vi "Write Configuration File.vi"(8 "error in (no error)":errorcluster, 11 "Example Instrument in":refnum<class "Instrument.LN2.lvclass">) -> (0 "error out":errorcluster, 3 "Example Instrument out":refnum<class "Instrument.LN2.lvclass">)   [LabVIEW 2019, in "Instrument.LN2.lvclass"]
uses:
  Instrument.LN2.lvclass
  <userlib>/LevyLab/Instrument Framework/Instrument Types/VSource/Instrument.VSource.lvclass
  <userlib>/LevyLab/Instrument Framework/SMOs/Configuration/Configuration.lvclass
  <userlib>/LevyLab/Instrument Framework/SMOs/Instrument/Instrument.lvclass
  C:/Program Files (x86)/National Instruments/LabVIEW 2019/user.lib/LevyLab/Instrument Framework/SMOs/Instrument/Instrument.lvclass
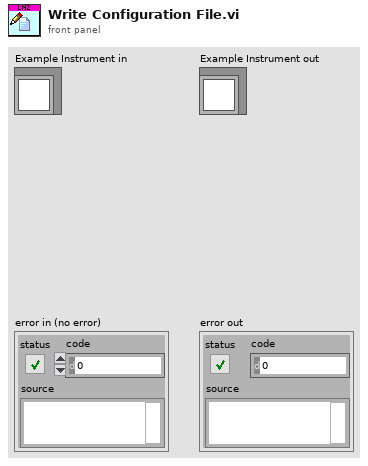
[diagram p1: front panel]
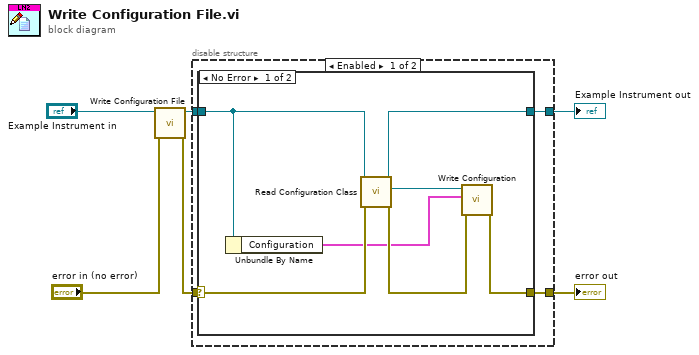
[diagram p0: block diagram]
diagram:
  n1 = call-parent "Write Configuration File.vi"("error in (no error)"="error in (no error)", "Instrument in"="Example Instrument in") -> ("error out"=w1:errorcluster, "Instrument out"=w2:refnum<class "Instrument.LN2.lvclass">)  [unwired: 8 in]
  n2 = disable-structure shown="Enabled" {
    disable-tunnel: [w10 w21] -> w6
    disable-tunnel: [w9 w20] -> w5
    disable-tunnel: w2 -> [w8 w21]
    disable-tunnel: w1 -> [w7 w20]
    frame Enabled {
      n3 = case shown="No Error" w7 {
        selector: w7 -> [w13 w19]
        tunnel: w8 -> [w12 w18]
        tunnel: [w16 w18] -> w10
        tunnel: [w15 w19] -> w9
        frame No Error {
          n4 = Unbundle By Name(w12) -> ("Configuration"=w11:cluster{"Fridge":string})
          n5 = call <userlib>:"Read Configuration Class.vi"("error in (no error)"=w13, "Instrument in"=w12) -> ("error out"=w17:errorcluster, "Configuration"=w14:refnum<class "Configuration.lvclass">, "Instrument out"=w16:refnum<class "Instrument.LN2.lvclass">)  [unwired: 7 in]
          n6 = call <userlib>:"Write Configuration.vi"("error in (no error)"=w17, "Variant"=w11, "Configuration in"=w14) -> ("error out"=w15:errorcluster)  [unwired: 7 in, 1 out]
        }
        frame Error {
        }
      }
    }
    frame Disabled {
    }
  }
  "Example Instrument out" <- w6
  "error out" <- w5
